vi "Waveform Gen.vi"() -> ()   [LabVIEW 2014]
panel:
  in  "Freq Multiplier":dbl(slide) scale=0.0..1.0
  in  "Stop":bool
  in  "Sine Amplitude":dbl(slide) scale=0.0..2.5
  in  "AO 1 Amplitude":dbl(slide) scale=0.0..5.0
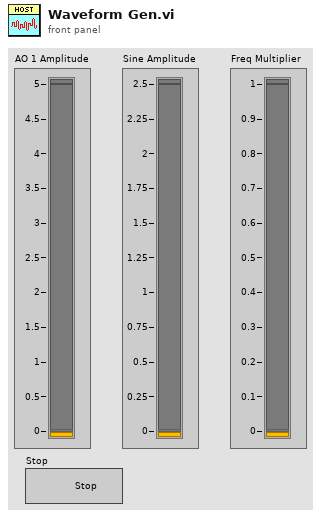
[diagram p1: front panel]
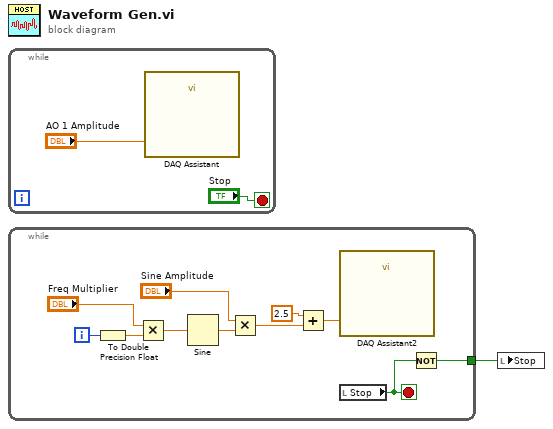
[diagram p0: block diagram]
diagram:
  n1 = while {
    stop <- "Stop" stop-if-true
    n2 = call "DAQ Assistant"("data"="AO 1 Amplitude") -> ()  [unwired: 17 in, 2 out]
  }
  n3 = while {
    tunnel: [w5] -> w1
    i -> [w13]
    stop <- w6 stop-if-true
    n4 = To Double Precision Float(number=w13) -> (double precision float=w8:dbl)
    n5 = Multiply(x="Freq Multiplier", y=w8) -> (x*y=w9:dbl)
    n6 = Sine(x=w9) -> (sin(x)=w14:dbl)
    n7 = Multiply(x="Sine Amplitude", y=w14) -> (x*y=w10:dbl)
    n8 = Add(x=2.5, y=w10) -> (x+y=w11:dbl)
    n9 = call "DAQ Assistant2"("data"=w11) -> ()  [unwired: 17 in, 2 out]
    n10 = local read "Stop"() -> (w6:bool)
    n11 = Not(x=w6) -> (.not. x?=w5:bool)
  }
  n12 = local write "Stop"(w1) -> ()
